vi "System Semaphore Destroy Handle.vi"(8 "error in (no error)":errorcluster, 11 "SemaphoreHandle":u16 format="%.0x") -> (0 "error out":errorcluster)   [LabVIEW 2011]
uses:
  kernel32.dll
panel:
  out "ERR DOE":u8
  # "This VI doesn't work yet, there's a problem with \nAccess rights. Destroy isn't really necessary since\nHandles are destroyed when the process that owns\nthem quits. The VI is currently disabled and harmless."
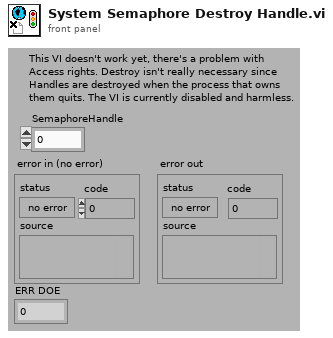
[diagram p1: front panel]
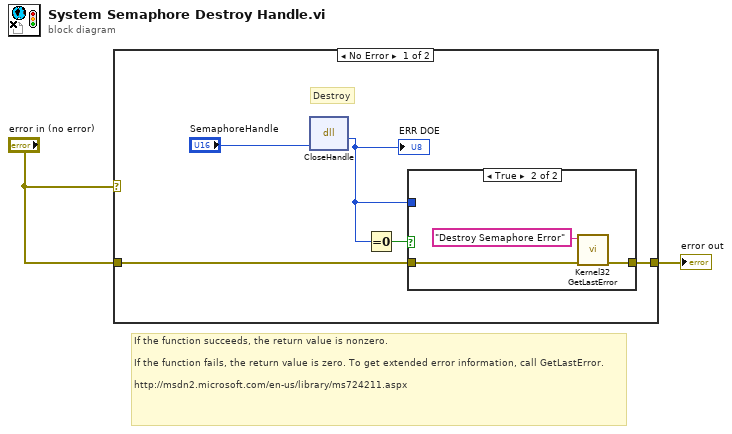
[diagram p0: block diagram]
diagram:
  # "If the function succeeds, the return value is nonzero.\n\nIf the function fails, the return value is zero. To get extended error information, call GetLastError.\n\nhttp://msdn2.microsoft.com/en-us/library/ms724211.aspx"
  n1 = case shown="No Error" "error in (no error)" {
    tunnel: "error in (no error)" -> [w5 w12]
    tunnel: [w4 w12] -> w2
    frame No Error {
      # "Destroy"
      n2 = dll-call lib="kernel32.dll" fn="CloseHandle"("SemaphoreHandle"="SemaphoreHandle") -> ("return type"=w3:u8)  [unwired: 4 in, 2 out]
      "ERR DOE" <- w3
      n3 = Equal To 0?(x=w3) -> (x = 0?=w6:bool)
      n4 = case shown="True" w6 {
        tunnel: w5 -> [w8 w11]
        tunnel: [w8 w10] -> w4
        tunnel: w3 -> [_ _]
        frame False {
        }
        frame True {
          n5 = call "Kernel32 GetLastError.vi"("error in (no error)"=w11, "Message"="Destroy Semaphore Error" ("source")) -> ("error out"=w10:errorcluster)  [unwired: 9 in]
        }
      }
    }
    frame Error {
    }
  }
  "error out" <- w2
